vi "SQLite Select Template.vi"(8 "error in":errorcluster, 10 "PK":cluster{}, 11 "SQLite Connection in":refnum<class "Connection.lvclass">) -> (0 "error out":errorcluster, 2 "Data":cluster{}, 3 "SQLite Connection out":refnum<class "Connection.lvclass">)   [LabVIEW 2021]
uses:
  <vilib>/drjdpowell/SQLite Library/SQL Statement/SQL Statement.lvclass
  <vilib>/drjdpowell/SQLite Library/SQL Connection/Connection.lvclass
  edt.lib/sqlite.lib/EDT SQLite+.lvlib
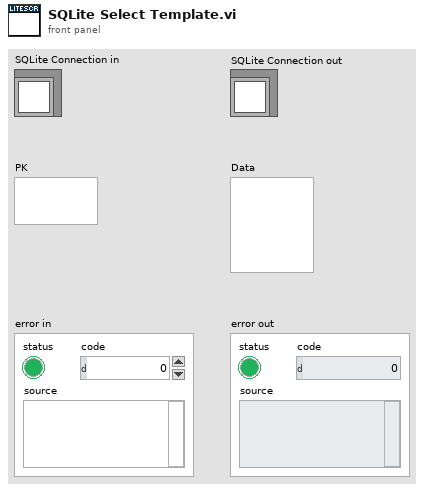
[diagram p1: front panel]
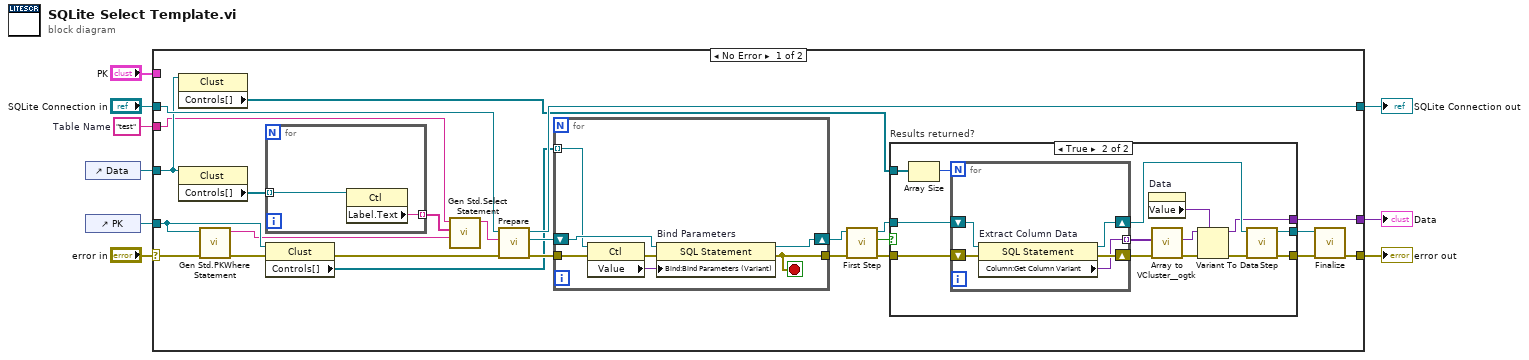
[diagram p0: block diagram]
diagram:
  w4 = "test"  # Table Name
  n1 = control-ref of="Data"() -> (w1:refnum<vi>)
  n2 = control-ref of="PK"() -> (w3:refnum<vi>)
  n3 = case shown="No Error" "error in" {
    selector: "error in" -> [w21 w66]
    tunnel: [w25 w66] -> w8
    tunnel: "PK" -> [_ _]
    tunnel: [w22 _] -> w2
    tunnel: "SQLite Connection in" -> [w24 w65]
    tunnel: [w23 w65] -> w5
    tunnel: w4 -> [w13 _]
    tunnel: w3 -> [w20 _]
    tunnel: w1 -> [w16 _]
    frame No Error {
      n4 = property on="Property Node" class="Clust"(reference=w16) -> ("Controls[]"=w15:refnum<vi>[])  [unwired: 1 in, 2 out]
      n5 = property on="Property Node" class="Clust"(reference=w16) -> ("Controls[]"=w14:refnum<vi>[])  [unwired: 1 in, 2 out]
      n6 = call "Gen Std.PKWhere Statement.vi"("error in"=w21, "Cluster in"=w20) -> ("error out"=w18:errorcluster, "delimited string"=w11:string)  [unwired: 8 in]
      n7 = for {
        tunnel: w14 -> [w36] mode=indexing
        tunnel: [w35] -> w12 mode=indexing
        n8 = property class="Ctl"(reference=w36) -> ("Label.Text"=w35:string)  [unwired: 1 in, 2 out]
      }
      n9 = property on="Property Node" class="Clust"(reference=w20, error in=w18) -> (error out=w17:errorcluster, "Controls[]"=w19:refnum<vi>[])  [unwired: 1 out]
      n10 = call "Gen Std.Select Statement.vi"("Filter String"=w11, "Fields"=w12, "Table Name"=w13) -> ("String"=w10:string)  [unwired: 8 in]
      n11 = call <vilib>:"Prepare.vi"("error in (no error)"=w17, "SQL"=w10, "SQLite Connection in"=w24) -> ("error out"=w32:errorcluster, "SQL Statement"=w29:refnum<class "SQL Statement.lvclass">, "SQLite Connection"=w23:refnum<class "Connection.lvclass">)  [unwired: 4 in, 2 out]
      n12 = for {
        shift-right: [w43] -> w30
        shift-left: w29 -> [w42]
        tunnel: w19 -> [w41] mode=indexing
        tunnel: w32 -> [w39]
        tunnel: [w37] -> w31
        stop <- w37 stop-if-true
        n13 = property class="Ctl"(reference=w41, error in=w39) -> (error out=w38:errorcluster, "Value"=w40:variant)  [unwired: 1 out]
        n14 = property on="Bind Parameters" class="SQL Statement"(reference=w42, error in=w38, "Bind:Bind Parameters (Variant)"=w40) -> (reference out=w43:refnum<class "SQL Statement.lvclass">, error out=w37:errorcluster)
      }
      n15 = call <vilib>:"First Step.vi"("error in (no error)"=w31, "SQL Statement in"=w30) -> ("error out"=w27:errorcluster, "Row returned"=w26:bool, "SQL Statement"=w28:refnum<class "SQL Statement.lvclass">)  [unwired: 7 in]
      n16 = case "Results returned?" shown="True" w26 {
        tunnel: [w45 w59] -> w33
        tunnel: [w44 w58] -> w34
        tunnel: w28 -> [w45 w57]
        tunnel: w27 -> [w44 w56]
        tunnel: [_ w53] -> w22
        tunnel: w15 -> [_ w50]
        frame False {
        }
        frame True {
          n17 = Array Size(array=w50) -> (size(s)=w51:i32)
          n18 = for {
            N: w51 -> [_]
            shift-right: [w64] -> w55
            shift-left: w57 -> [w63]
            shift-right: [w61] -> w47
            shift-left: w56 -> [w62]
            tunnel: [w60] -> w49 mode=indexing
            n19 = property on="Extract Column Data" class="SQL Statement"(reference=w63, error in=w62) -> (reference out=w64:refnum<class "SQL Statement.lvclass">, error out=w61:errorcluster, "Column:Get Column Variant"=w60:variant)
          }
          n20 = property on="Data" class="Clust"() -> ("Value"=w54:variant)  [unwired: 2 in, 2 out]
          n21 = call <userlib>:"Array to VCluster__ogtk.vi"("error in (no error)"=w47, "Array"=w49) -> ("error out"=w48:errorcluster, "VCluster"=w46:variant)  [unwired: 8 in]
          n22 = Variant To Data(error in=w48, type=w54, Variant=w46) -> (data=w53:variant, error out=w52:errorcluster)
          n23 = call <vilib>:"Step.vi"("error in (no error)"=w52, "SQL Statement in"=w55) -> ("error out"=w58:errorcluster, "SQL Statement"=w59:refnum<class "SQL Statement.lvclass">)  [unwired: 7 in, 1 out]
        }
      }
      n24 = call <vilib>:"Finalize.vi"("error in (no error)"=w34, "SQL Statement in"=w33) -> ("error out"=w25:errorcluster)  [unwired: 9 in]
    }
    frame Error {
    }
  }
  "error out" <- w8
  "Data" <- w2
  "SQLite Connection out" <- w5
